vi "sm.init.vi"   [LabVIEW 2019]
uses:
  <vilib>/rvi/Emulation/niFpgaEmulationIsFPGAContextNoSignature.vi
  <vilib>/rvi/DataTransferAndStorage/Container/Common/niFpgaContainerGetUniqueNameForEmu.vi
  <vilib>/rvi/Memory/Memory_Emulation/niFpgaMemoryEmulationCacheClearOnFirstRun.vi
  <vilib>/rvi/Memory/Memory_Emulation/nirvimemoryEmulationManagerCache_MakeExclusive.vi
  <vilib>/rvi/Memory/Memory_Emulation/niFpgaMemoryEmulationValidateCache.vi
  <vilib>/rvi/Memory/Memory_Emulation/nirvimemoryEmulationManagerCache_InsertValue.vi
  <vilib>/Utility/error.llb/Clear Errors.vi
  <vilib>/rvi/Memory/Memory_Emulation/nirvimemoryEmulationManagerCache_ReleaseExclusive.vi
  <vilib>/rvi/Memory/Memory_Emulation/nirvimemoryEmulationManagerCache_GetValue.vi
  <vilib>/rvi/Memory/Memory_Emulation/nirvimemoryEmulationManagerCache_SetValue.vi
  <vilib>/rvi/Emulation/niFpgaProcessEmulError.vi
  <vilib>/rvi/Emulation/niFpgaSctlEmulationGetInTimedLoop.vi
  <vilib>/rvi/DataTransferAndStorage/Container/XNode/niFpgaContainer.xnode
  <vilib>/rvi/DataTransferAndStorage/Register/Emulation/niFpgaRegisterEmulation.vi
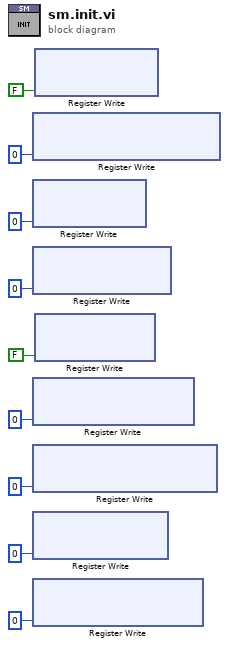
[diagram p0: block diagram]
diagram:
  n1 = xnode "Register Write"("Data"=u32 0) -> ()  [unwired: 1 in, 1 out]
  n2 = xnode "Register Write"("Data"=u8 0) -> ()  [unwired: 1 in, 1 out]
  n3 = xnode "Register Write"("Data"=u8 0) -> ()  [unwired: 1 in, 1 out]
  n4 = xnode "Register Write"("Data"=u32 0) -> ()  [unwired: 1 in, 1 out]
  n5 = xnode "Register Write"("Data"=u32 0) -> ()  [unwired: 1 in, 1 out]
  n6 = xnode "Register Write"("Data"=u8 0) -> ()  [unwired: 1 in, 1 out]
  n7 = xnode "Register Write"("Data"=u32 0) -> ()  [unwired: 1 in, 1 out]
  n8 = xnode "Register Write"("Data"=FALSE) -> ()  [unwired: 1 in, 1 out]
  n9 = xnode "Register Write"("Data"=FALSE) -> ()  [unwired: 1 in, 1 out]
